vi "Parse GSA.vi"(8 "error in (no error)":errorcluster, 10 "Message":refnum<class "NMEA Message.lvclass">, 11 "nmea in":refnum<class "nmea.lvclass">) -> (0 "error out":errorcluster, 3 "nmea out":refnum<class "nmea.lvclass">)   [LabVIEW 2020, in "nmea.lvlib" / "nmea.lvclass"]
uses:
  nmea.lvclass
  message/NMEA Message.lvclass
  GSA Field.ctl
  nmea.lvclass/nmea.ctl
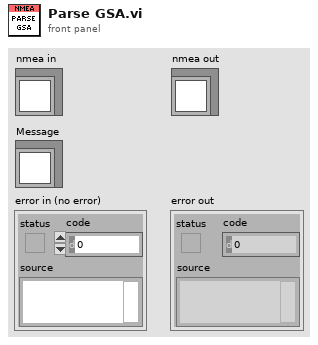
[diagram p1: front panel]
types:
  T1 = typedef "nmea.lvlib/nmea.lvclass/GSA Field.ctl" = enum16{"Mode", "Fix", "SV 1", "SV 2", "SV 3", "SV 4", "SV 5", "SV 6", "SV 7", "SV 8", "SV 9", "SV 10", "SV 11", "SV 12", "PDOP", "HDOP", "VDOP"}
  T2 = typedef "nmea.lvlib/nmea.lvclass/Fix Mode.ctl" = enum16{"Manual", "Auto 2/3D"}
  T3 = typedef "nmea.lvlib/nmea.lvclass/Fix Type.ctl" = enum16{"N/A", "None", "2D", "3D"}
  T4 = typedef "nmea.lvlib/nmea.lvclass/Ref Data.ctl" = cluster{"Latitude":dbl, "Longitude":dbl, "Time":T5, "Status":string, "Speed":dbl, "Course":dbl, "Mag Var":dbl, "Var Dir":string, "Mode":string, "Satellites":T6[], "Next Satellites":T6[], "Active PRNs":i32[], "Fix Type":T3, "DOP":T7, "Fix Mode":T2, "Altitude":dbl, "Geoid":dbl}
  T5 = typedef "LVDateTimeRec.ctl" = cluster{"fractional second":dbl, "second":i32, "minute":i32, "hour":i32, "day of month":i32, "month":i32, "year":i32, "day of week":i32, "day of year":i32, "DST":i32}
  T6 = typedef "nmea.lvlib/nmea.lvclass/Satellite.ctl" = cluster{"PRN":u8, "Channel":u8, "Elevation":u8, "Azimuth":u16, "SNR":u8, "Active":bool}
  T7 = typedef "nmea.lvlib/nmea.lvclass/DOP.ctl" = cluster{"P":dbl, "H":dbl, "V":dbl}
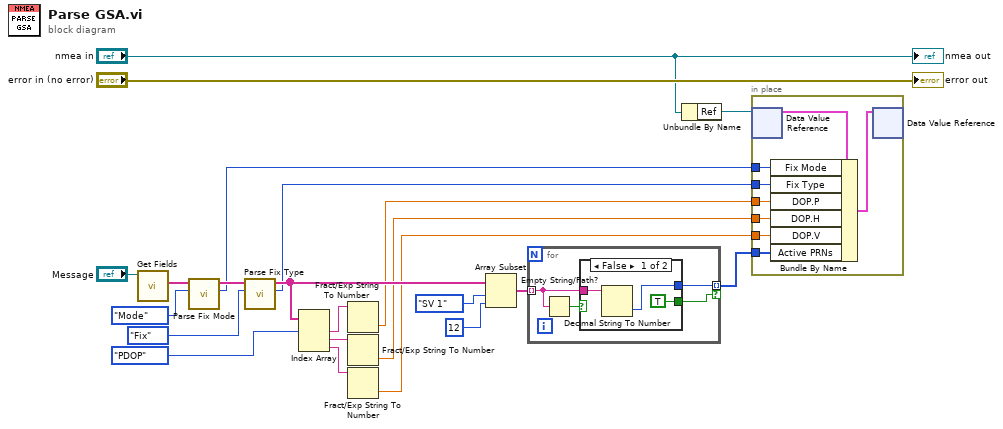
[diagram p0: block diagram]
diagram:
  n1 = call "Get Fields.vi"("NMEA Message in"="Message") -> ("Fields"=w4:string[])  [unwired: 8 in, 2 out]
  n2 = call "Parse Fix Mode.vi"("Mode Index"=GSA_Field."Mode" ("GSA Fields"), "Fields In"=w4) -> ("Fix Mode"=w1:T2, "Fields"=w3:string[])  [unwired: 8 in]
  n3 = call "Parse Fix Type.vi"("Fix Index"=GSA_Field."Fix" ("GSA Fields"), "Fields In"=w3) -> ("Fix Type"=w9:T3, "Fields"=w15:string[])  [unwired: 8 in]
  n4 = Index Array(array=w15, index #1=GSA_Field."PDOP" ("GSA Fields")) -> (element #1=w17:string, element #2=w18:string, element #3=w16:string)  [unwired: 2 in]
  n5 = Fract/Exp String To Number(string=w17) -> (number=w8:dbl)  [unwired: 3 in, 1 out]
  n6 = Fract/Exp String To Number(string=w18) -> (number=w7:dbl)  [unwired: 3 in, 1 out]
  n7 = Fract/Exp String To Number(string=w16) -> (number=w6:dbl)  [unwired: 3 in, 1 out]
  n8 = Array Subset(array=w15, index=GSA_Field."SV 1" ("GSA Fields"), length=12) -> (w12:string[])
  n9 = for {
    tunnel: w12 -> [w25] mode=indexing
    tunnel: [w24] -> w5 mode=indexing if=w23
    n10 = Empty String/Path?(string/path=w25) -> (empty?=w26:bool)
    n11 = case shown="False" w26 {
      tunnel: w25 -> [w29 _]
      tunnel: [w28 _] -> w24
      tunnel: [TRUE _] -> w23
      frame False {
        n12 = Decimal String To Number(string=w29) -> (number=w28:i32)  [unwired: 2 in, 1 out]
      }
      frame True {
      }
    }
  }
  n13 = Unbundle By Name("nmea in") -> ("Ref"=w11:refnum<data-value>)
  n14 = in-place {
    in-place-border: w9 -> [w35]
    in-place-border: w8 -> [w34]
    in-place-border: w7 -> [w33]
    in-place-border: w6 -> [w32]
    in-place-border: w5 -> [w31]
    in-place-border: w1 -> [w30]
    n15 = in-place-dvr #1(w11) -> (w37:T4)  [unwired: 1 out]
    n16 = Bundle By Name(cluster=w37, "Fix Mode"=w30, "Fix Type"=w35, "DOP.P"=w34, "DOP.H"=w33, "DOP.V"=w32, "Active PRNs"=w31) -> (w36:T4)
    n17 = in-place-dvr #1(w36) -> ()  [unwired: 2 out]
  }
  "error out" <- "error in (no error)"
  "nmea out" <- "nmea in"
